vi "Helm Send Status.vi"(8 "error in (no error)":errorcluster, 11 "RDS Helm Actor in":refnum<class "RDS Helm Actor.lvclass">) -> (0 "error out":errorcluster, 3 "RDS Helm Actor out":refnum<class "RDS Helm Actor.lvclass">)   [LabVIEW 2015, in "RDS Helm Actor.lvlib" / "RDS Helm Actor.lvclass"]
uses:
  RDS Helm Actor.lvclass
  Libraries/RDS Child Messages/Helm/Helm Status Message/Helm Status Message.lvclass
  Libraries/RDS Framework/RDS Message ID.ctl
  Libraries/RDS Child Messages/Helm/Helm Status Message/Helm Status Control.ctl
  Helm State.ctl
  Libraries/RDS Child Messages/Helm/Heading Command/Heading Command Cntrl.ctl
  Libraries/RDS Child Messages/Helm/Steering Command/Steering Command Cntrl.ctl
  Libraries/RDS Child Messages/PID Gains/PID Gains Control.ctl
  RDS Helm Actor.lvclass/RDS Helm Actor.ctl
  Libraries/RDS Framework/RDS Message Class/RDS Message.lvclass/RDS Message.ctl
  Libraries/RDS Child Messages/Helm/Helm Status Message/Helm Status Message.lvclass/Helm Status Message.ctl
  Libraries/RDS Framework/RDS Message Class/RDS Message.lvclass
  Libraries/RDS Child Messages/RDS Child Messages.lvlib
  RDS Helm Actor.lvlib
  RDS Parent Actor/RDS Parent Actor/RDS Parent Actor.lvclass
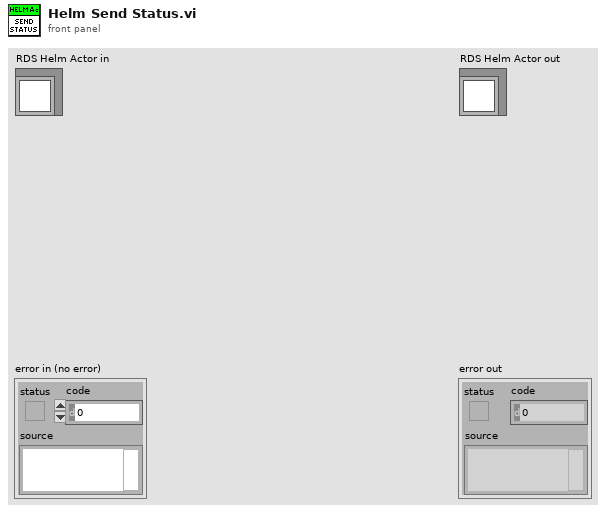
[diagram p1: front panel]
types:
  T1 = typedef "RDS Child Messages.lvlib/Helm Status Control.ctl" = cluster{"Helm State":T2, "Heading Command Control":T3, "Steering Command Control":T4, "Last Command Time":timestamp, "Gains":T5, "Current Heading":dbl, "Port Throttle":i16, "STBD Throttle":i16, "Limiter":dbl}
  T2 = typedef "RDS Helm Actor.lvlib/Helm State.ctl" = enum16{"Idle", "Executing Heading Command", "Executing Steering Command"}
  T3 = typedef "RDS Child Messages.lvlib/Heading Command Cntrl.ctl" = cluster{"Throttle":i16, "Heading":sgl, "Duration (s)":i16}
  T4 = typedef "RDS Child Messages.lvlib/Steering Command Cntrl.ctl" = cluster{"Throttle":i16, "Rudder":i8, "Duration (s)":u16}
  T5 = typedef "RDS Child Messages.lvlib/PID Gains Control.ctl" = cluster{"P (Kc)":sgl, "I (Ti)":sgl, "D (Td)":sgl}
  T6 = typedef "RDS Child Messages.lvlib/RDS Message ID.ctl" = enum16{"RDS Hello World", "String Message", "AIP_Status", "AIP_Command", "GPS_Data", "MCB_Command", "MCB_Status", "Compass_Data", "Depth_Data", "Battery_Data", "Contoller_State", "Set_Mag_Dev", "BTB_Shutdown", "State_Sample_Request", "State_Sample", "PID_Gains_Set", "Helm_Limiter_Set", "Helm_Heading_Command", "Helm_Steering_Command", "Helm_Status", "Controller_Message", "AIP_Set_Min_Depth", "Mission_Controller_State", "Mission_Upload", "Mission_Set_Op_and_Run", "Mission_Settings_Set"}
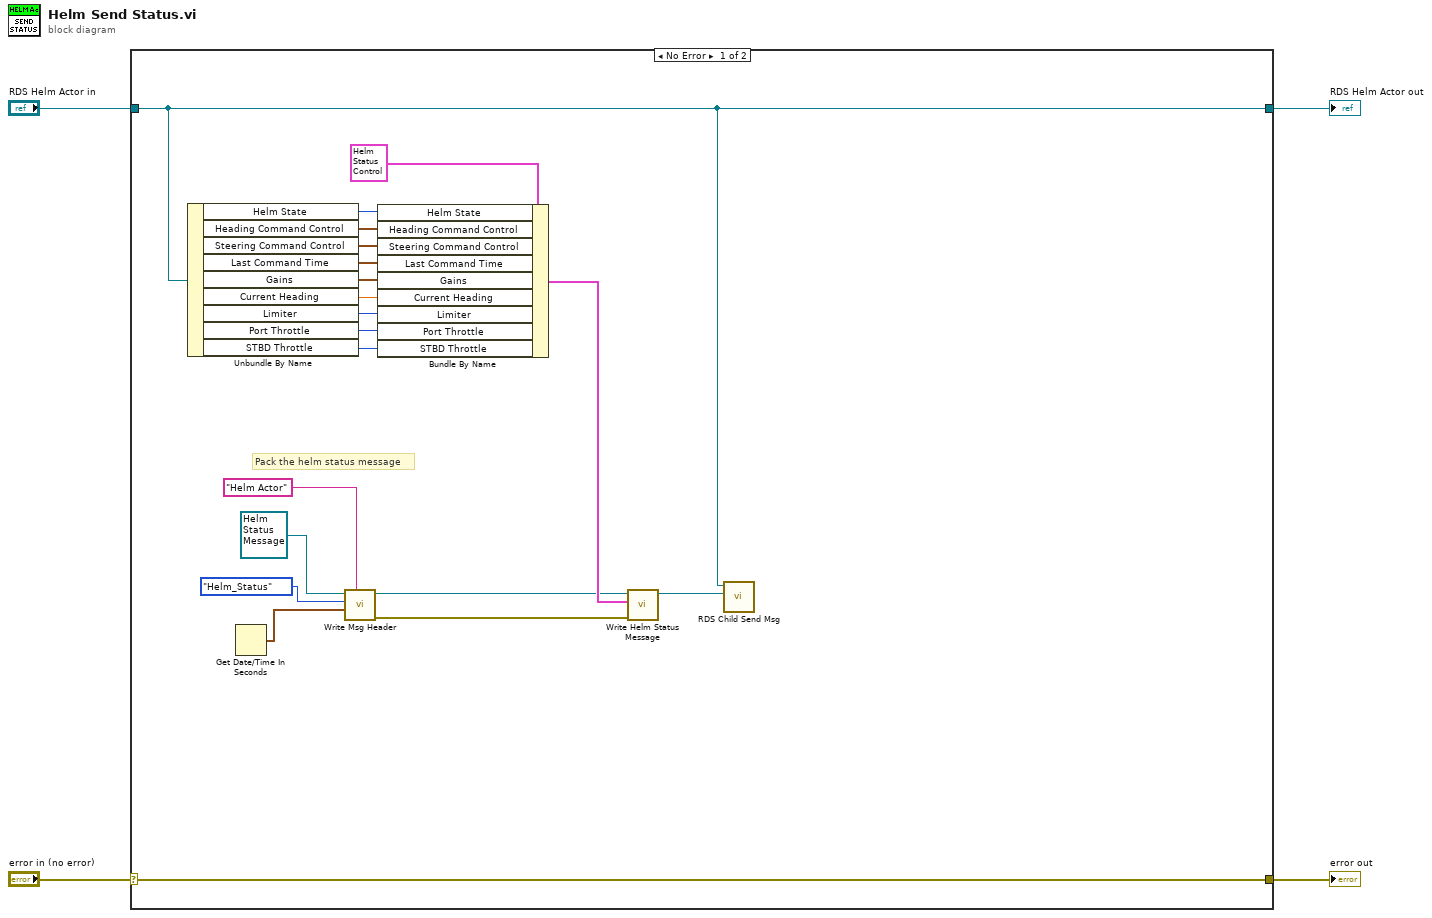
[diagram p0: block diagram]
diagram:
  n1 = case shown="No Error" "error in (no error)" {
    selector: "error in (no error)" -> [w24 w26]
    tunnel: [w24 w26] -> w3
    tunnel: [w8 w25] -> w1
    tunnel: "RDS Helm Actor in" -> [w8 w25]
    frame No Error {
      # "Pack the helm status message"
      n2 = Unbundle By Name(w8) -> ("Helm State"=w18:T2, "Heading Command Control"=w17:T3, "Steering Command Control"=w16:T4, "Last Command Time"=w15:timestamp, "Gains"=w14:T5, "Current Heading"=w13:sgl, "Limiter"=w7:u8, "Port Throttle"=w6:i16, "STBD Throttle"=w5:i16)
      n3 = Get Date/Time In Seconds() -> (seconds since 1Jan1904=w23:timestamp)
      n4 = call "Write Msg Header.vi"("Sender Name"="Helm Actor", "Time Stamp"=w23, "Msg ID"=RDS_Message_ID."Helm_Status", "RDS Message in"=refnum<class "Helm Status Message.lvclass"> refnum ("RDS Child Messages.lvlib:Helm Status Message.lvclass")) -> ("error out"=w10:errorcluster, "RDS Message out"=w11:refnum<class "Helm Status Message.lvclass">)  [unwired: 6 in]
      n5 = Bundle By Name(cluster=T1 {"Helm State"=enum."Idle", "Heading Command Control"={"Throttle"=0, "Heading"=0.0, "Duration (s)"=0}, "Steering Command Control"={"Throttle"=0, "Rudder"=0, "Duration (s)"=0}, "Last Command Time"=timestamp(0 s since 1904-01-01), "Gains"={"P (Kc)"=0.0, "I (Ti)"=0.0, "D (Td)"=0.0}, "Current Heading"=0.0, "Port Throttle"=0, "STBD Throttle"=0, "Limiter"=0.0} ("Helm Status"), "Helm State"=w18, "Heading Command Control"=w17, "Steering Command Control"=w16, "Last Command Time"=w15, "Gains"=w14, "Current Heading"=w13, "Limiter"=w7, "Port Throttle"=w6, "STBD Throttle"=w5) -> (w12:T1)
      n6 = call "Write Helm Status Message.vi"("error in (no error)"=w10, "Helm Status"=w12, "Helm Status Message in"=w11) -> ("Helm Status Message out"=w9:refnum<class "Helm Status Message.lvclass">)  [unwired: 7 in, 1 out]
      n7 = call "RDS Child Send Msg.vi"("RDS Message"=w9, "RDS Parent Actor in"=w8) -> ()  [unwired: 8 in, 2 out]
    }
    frame Error {
    }
  }
  "error out" <- w3
  "RDS Helm Actor out" <- w1
